vi "FittedCircle.vi"(7 "pts":i32=100, 9 "r":dbl, 11 "x0, y0, z0":dbl[](array[numeric]) format="%.2f") -> (2 "Y":dbl[](array[numeric]), 3 "X":dbl[](array[numeric]))   [LabVIEW 2022 SP3]
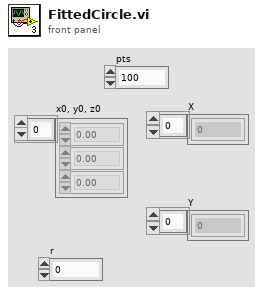
[diagram p1: front panel]
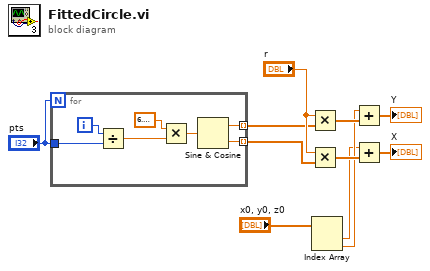
[diagram p0: block diagram]
diagram:
  n1 = for {
    N: "pts" -> [_]
    tunnel: "pts" -> [w17]
    tunnel: [w14] -> w5 mode=indexing
    tunnel: [w13] -> w7 mode=indexing
    i -> [w18]
    n2 = Divide(x=w18, y=w17) -> (x/y=w16:dbl)
    n3 = Multiply(x=6.283185307179586, y=w16) -> (x*y=w12:dbl)
    n4 = Sine & Cosine(0:w12) -> (1:w14:dbl, 2:w13:dbl)
  }
  n5 = Multiply(x="r", y=w5) -> (x*y=w8:dbl[])
  n6 = Multiply(x="r", y=w7) -> (x*y=w10:dbl[])
  n7 = Index Array(array="x0, y0, z0") -> (element #1=w1:dbl, element #2=w2:dbl)  [unwired: 2 in]
  n8 = Add(x=w2, y=w8) -> (x+y=→"Y":dbl[])
  n9 = Add(x=w1, y=w10) -> (x+y=→"X":dbl[])
